vi "Bot.vi"(7 "BotData":T3, 11 "GameState":T1) -> (0 "error out":errorcluster, 3 "Move":T4)   [LabVIEW 2015, in "StraightBot.lvlib"]
uses:
  StraightBot.lvlib
  TronVIEWBotAPI/MovementDirection.ctl
  TronVIEWBotAPI/BotData.ctl
  TronVIEWBotAPI/GameState.ctl
  TronviewGame/Board/Position.ctl
  <vilib>/Analysis/1siggen.llb/Riffle Array (I32).vi
  TronVIEWGameUtilities/TronVIEWGameUtilities.lvlib
  TronVIEWBotAPI/TronVIEWBotAPI.lvlib
  <vilib>/Analysis/NI_AALBase.lvlib
  TronviewGame/Board/Board.lvclass
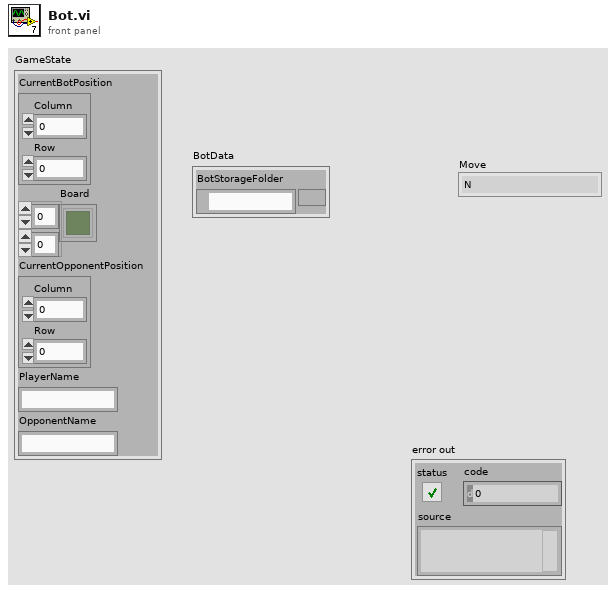
[diagram p1: front panel]
types:
  T1 = typedef "TronVIEWBotAPI.lvlib/GameState.ctl" = cluster{"CurrentBotPosition":T2, "Board":bool[][], "CurrentOpponentPosition":T2, "PlayerName":string, "OpponentName":string}
  T2 = typedef "TronviewGame.lvlib/Board.lvclass/Position.ctl" = cluster{"Column":i32, "Row":i32}
  T3 = typedef "TronVIEWBotAPI.lvlib/BotData.ctl" = cluster{"BotStorageFolder":path}
  T4 = typedef "TronVIEWBotAPI.lvlib/MovementDirection.ctl" = enum16{"N", "S", "W", "E"}
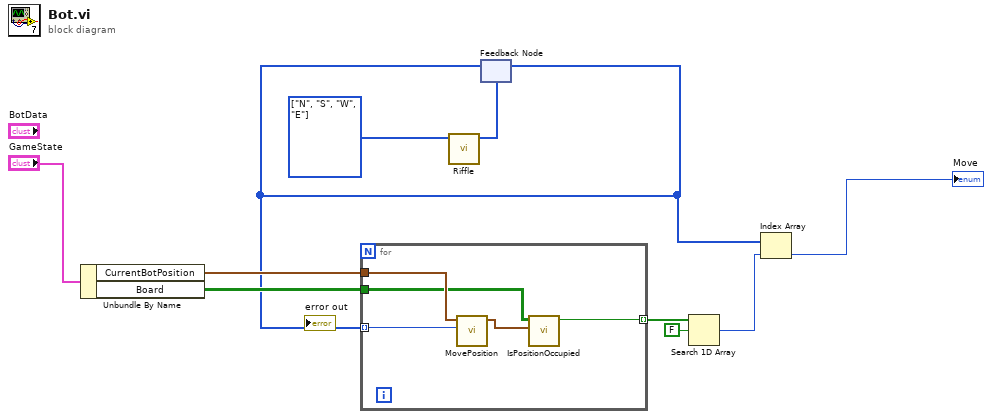
[diagram p0: block diagram]
diagram:
  w8 = T4[] [enum."N", enum."S", enum."W", enum."E"] items=["N", "S", "W", "E"]
  n1 = Unbundle By Name("GameState") -> ("CurrentBotPosition"=w10:T2, "Board"=w9:bool[][])
  n2 = call-poly <vilib>:"Riffle.vi"("X"=w8) -> ("Riffled {X}"=w6:i32[])  [unwired: 8 in, 2 out]
  n3 = feedback #1(w6) -> (w3:i32[])
  n4 = for {
    tunnel: w10 -> [w15]
    tunnel: w9 -> [w14]
    tunnel: w3 -> [w12] mode=indexing
    tunnel: [w11] -> w5 mode=indexing
    n5 = call "MovePosition.vi"("Direction"=w12, "PlayerPosition"=w15) -> ("NewPlayerPosition"=w13:T2)  [unwired: 9 in]
    n6 = call "IsPositionOccupied.vi"("Position"=w13, "Board"=w14) -> ("Occupied?"=w11:bool)  [unwired: 9 in]
  }
  n7 = feedback-in #1(w3) -> ()
  n8 = Search 1D Array(1D array=w5, element=FALSE) -> (index of element=w2:i32)  [unwired: 1 in]
  n9 = Index Array(array=w3, index=w2) -> (element=→"Move":i32)
